vi "SwerveReverseFeedback.vi"(9 "Invert Feedback Sensor":bool, 11 "Swerve Drive Param":T1(ring)) -> ()   [LabVIEW 2016]
uses:
  Robot Global Data.vi
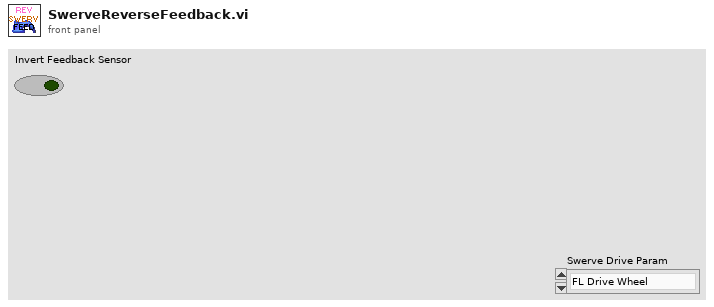
[diagram p1: front panel]
types:
  T1 = enum16{"FL Drive Wheel", "FR Drive Wheel", "RL Drive Wheel", "RR Drive Wheel", "FL Steer Wheel", "FR Steer Wheel", "RL Steer Wheel", "RR Steer Wheel"}
  T2 = typedef "WPI_DriverStationRobotMode2.ctl" = enum16{"Autonomous Disabled", "Autonomous Enabled", "Teleop Disabled", "Teleop Enabled", "Disconnected", "Finish", "Test Disabled", "Test Enabled", "Emergency Stopped"}
  T3 = typedef "WPI_CANTalonSRX_APIFeedbackSelect.ctl" = enum16{"Digital Quadrature Encoder", "Analog Potentiometer", "Analog Encoder", "Count on Quad-A (Rising-Edge)", "Count on Quad-A (Falling-Edge)", "CTR Magnetic Enc (Absolute)", "CTR Magnetic Enc (Relative)", "Pulse Width"}
  T4 = typedef "WPI_MotorControlDeviceRef.ctl" = cluster{"DeviceStatus":errorcluster, "Type":T5, "PWM":cluster{"PWM Channel":T6, "DeadBand":T7}, "CAN":cluster{"Device Number":u8, "SetOutput VI Ref":variant, "GetOutput VI Ref":variant, "Enable VI Ref":variant, "Disable VI Ref":variant, "Data":variant}, "Invert":bool}
  T5 = typedef "WPI_MotorControlType.ctl" = enum16{"PWM", "CAN"}
  T6 = typedef "FPGA_DIOPWMChannel.ctl" = enum8{"PWM 0", "PWM 1", "PWM 2", "PWM 3", "PWM 4", "PWM 5", "PWM 6", "PWM 7", "PWM 8", "PWM 9", "PWM MXP 0", "PWM MXP 1", "PWM MXP 2", "PWM MXP 3", "PWM MXP 4", "PWM MXP 5", "PWM MXP 6", "PWM MXP 7", "PWM MXP 8", "PWM MXP 9", "Invalid"}
  T7 = typedef "WPI_PWMDeadband.ctl" = cluster{"Name":string, "maxPositivePwm":i32, "minPositivePwm":i32, "centerPwm":i32, "maxNegativePwm":i32, "minNegativePwm":i32, "angularRange":u16}
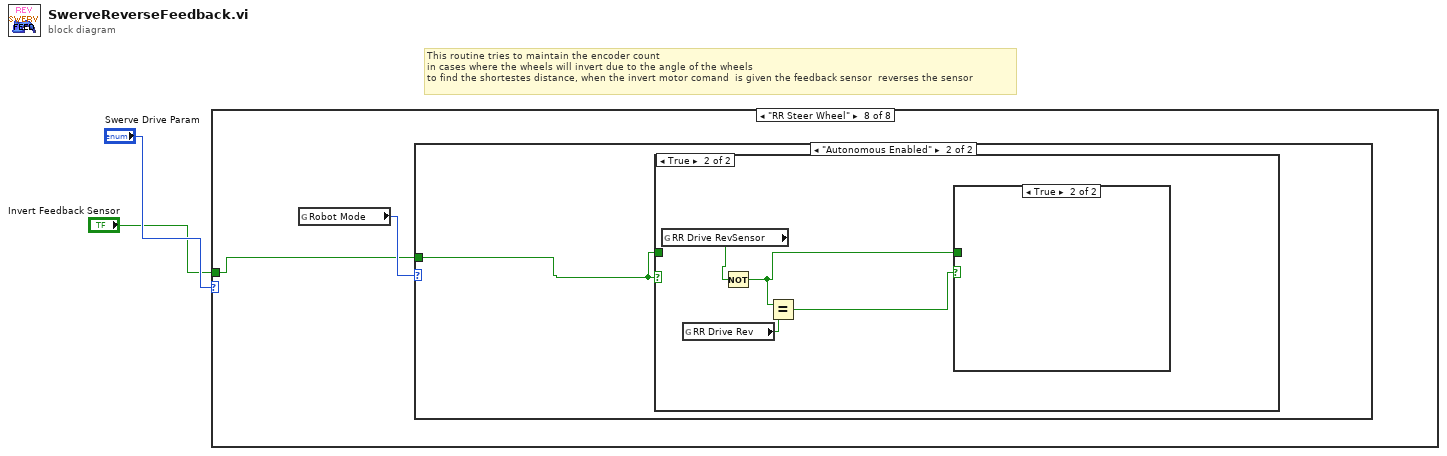
[diagram p0: block diagram]
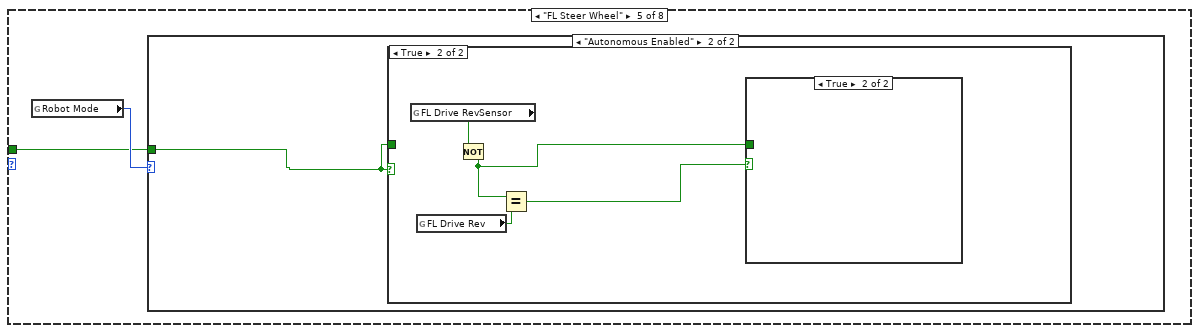
[diagram p6: hidden frame]
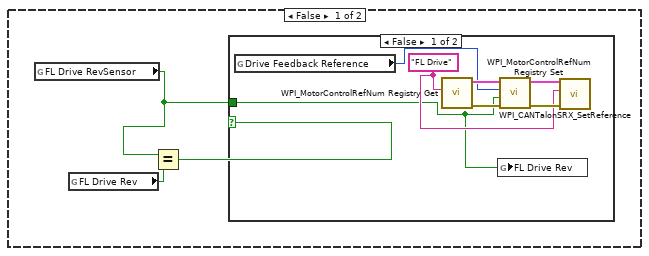
[diagram p8: hidden frame]
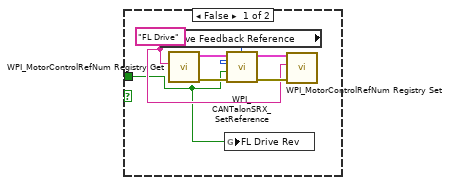
[diagram p10: hidden frame]
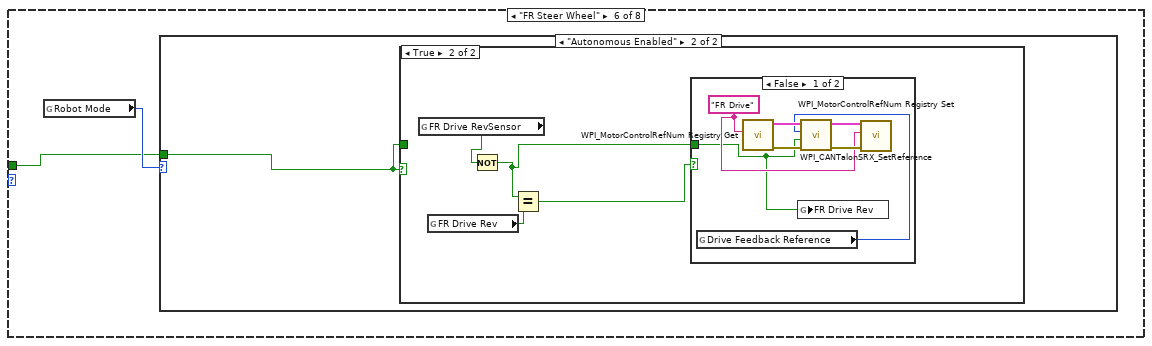
[diagram p11: hidden frame]
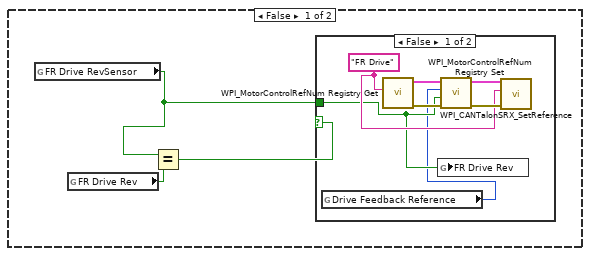
[diagram p13: hidden frame]
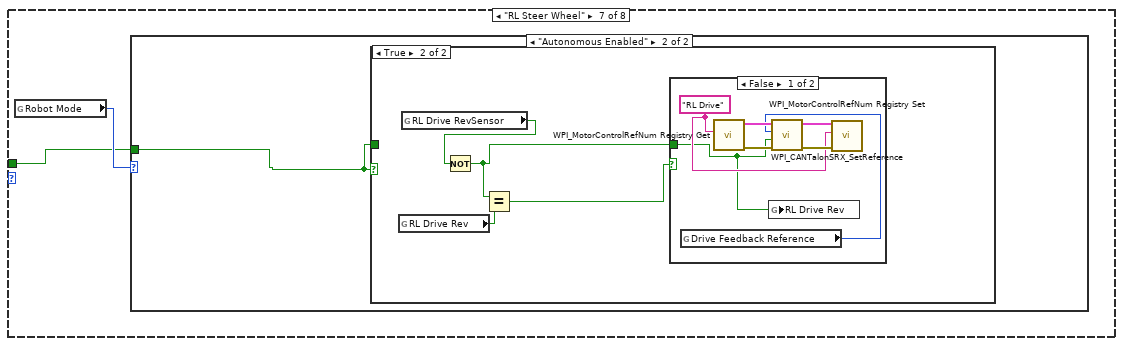
[diagram p16: hidden frame]
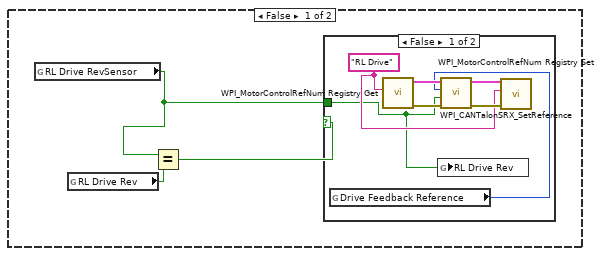
[diagram p18: hidden frame]
diagram:
  # "This routine tries to maintain the encoder count \nin cases where the wheels will invert due to the angle of the wheels \nto find the shortestes distance, when the invert motor comand  is given the feedback sensor  reverses the sensor"
  n1 = case shown="\"RR Steer Wheel\"" "Swerve Drive Param" {
    tunnel: "Invert Feedback Sensor" -> [_ _ _ _ w3 w27 w51 w75]
    frame "FL Drive Wheel", Default {
    }
    frame "FR Drive Wheel" {
    }
    frame "RL Drive Wheel" {
    }
    frame "RR Drive Wheel" {
    }
    frame "FL Steer Wheel" {
      n2 = global read "Robot Global Data.vi" "Robot Mode"() -> (w4:T2)
      n3 = case shown="\"Autonomous Enabled\"" w4 {
        tunnel: w3 -> [_ w5]
        frame "Autonomous Disabled", Default {
        }
        frame "Autonomous Enabled" {
          n4 = case shown="True" w5 {
            tunnel: w5 -> [_ _]
            frame False {
              n5 = global read "Robot Global Data.vi" "FL Drive RevSensor"() -> (w6:bool)
              n6 = global read "Robot Global Data.vi" "FL Drive Rev"() -> (w8:bool)
              n7 = Equal?(x=w6, y=w8) -> (x = y?=w7:bool)
              n8 = case shown="False" w7 {
                tunnel: w6 -> [w10 _]
                frame False {
                  w11 = "FL Drive" ("refnum name")
                  n9 = global read "Robot Global Data.vi" "Drive Feedback Reference"() -> (w9:T3)
                  n10 = call <vilib>:"WPI_MotorControlRefNum Registry Get.vi"("refnum name"=w11) -> ("error out"=w15:errorcluster, "MotorControlDevRef"=w14:T4)  [unwired: 9 in]
                  n11 = global write "Robot Global Data.vi" "FL Drive Rev"(w10) -> ()
                  n12 = call <vilib>:"WPI_CANTalonSRX_SetReference.vi"("error in (no error)"=w15, "Reverse Feedback Sensor"=w10, "Feedback Reference"=w9, "CAN Talon SRX Ref"=w14) -> ("error out"=w13:errorcluster, "CAN Talon SRX Ref"=w12:T4)  [unwired: 6 in]
                  n13 = call <vilib>:"WPI_MotorControlRefNum Registry Set.vi"("error in (no error)"=w13, "refnum name"=w11, "MotorControlDevRef"=w12) -> ()  [unwired: 7 in, 2 out]
                }
                frame True {
                }
              }
            }
            frame True {
              n14 = global read "Robot Global Data.vi" "FL Drive RevSensor"() -> (w17:bool)
              n15 = global read "Robot Global Data.vi" "FL Drive Rev"() -> (w19:bool)
              n16 = Not(x=w17) -> (.not. x?=w16:bool)
              n17 = Equal?(x=w16, y=w19) -> (x = y?=w18:bool)
              n18 = case shown="True" w18 {
                tunnel: w16 -> [w21 _]
                frame False {
                  w22 = "FL Drive" ("refnum name")
                  n19 = global read "Robot Global Data.vi" "Drive Feedback Reference"() -> (w20:T3)
                  n20 = call <vilib>:"WPI_MotorControlRefNum Registry Get.vi"("refnum name"=w22) -> ("error out"=w26:errorcluster, "MotorControlDevRef"=w25:T4)  [unwired: 9 in]
                  n21 = global write "Robot Global Data.vi" "FL Drive Rev"(w21) -> ()
                  n22 = call <vilib>:"WPI_CANTalonSRX_SetReference.vi"("error in (no error)"=w26, "Reverse Feedback Sensor"=w21, "Feedback Reference"=w20, "CAN Talon SRX Ref"=w25) -> ("error out"=w24:errorcluster, "CAN Talon SRX Ref"=w23:T4)  [unwired: 6 in]
                  n23 = call <vilib>:"WPI_MotorControlRefNum Registry Set.vi"("error in (no error)"=w24, "refnum name"=w22, "MotorControlDevRef"=w23) -> ()  [unwired: 7 in, 2 out]
                }
                frame True {
                }
              }
            }
          }
        }
      }
    }
    frame "FR Steer Wheel" {
      n24 = global read "Robot Global Data.vi" "Robot Mode"() -> (w28:T2)
      n25 = case shown="\"Autonomous Enabled\"" w28 {
        tunnel: w27 -> [_ w29]
        frame "Autonomous Disabled", Default {
        }
        frame "Autonomous Enabled" {
          n26 = case shown="True" w29 {
            tunnel: w29 -> [_ _]
            frame False {
              n27 = global read "Robot Global Data.vi" "FR Drive RevSensor"() -> (w30:bool)
              n28 = global read "Robot Global Data.vi" "FR Drive Rev"() -> (w32:bool)
              n29 = Equal?(x=w30, y=w32) -> (x = y?=w31:bool)
              n30 = case shown="False" w31 {
                tunnel: w30 -> [w34 _]
                frame False {
                  w35 = "FR Drive" ("refnum name")
                  n31 = global read "Robot Global Data.vi" "Drive Feedback Reference"() -> (w33:T3)
                  n32 = call <vilib>:"WPI_MotorControlRefNum Registry Get.vi"("refnum name"=w35) -> ("error out"=w39:errorcluster, "MotorControlDevRef"=w38:T4)  [unwired: 9 in]
                  n33 = global write "Robot Global Data.vi" "FR Drive Rev"(w34) -> ()
                  n34 = call <vilib>:"WPI_CANTalonSRX_SetReference.vi"("error in (no error)"=w39, "Reverse Feedback Sensor"=w34, "Feedback Reference"=w33, "CAN Talon SRX Ref"=w38) -> ("error out"=w37:errorcluster, "CAN Talon SRX Ref"=w36:T4)  [unwired: 6 in]
                  n35 = call <vilib>:"WPI_MotorControlRefNum Registry Set.vi"("error in (no error)"=w37, "refnum name"=w35, "MotorControlDevRef"=w36) -> ()  [unwired: 7 in, 2 out]
                }
                frame True {
                }
              }
            }
            frame True {
              n36 = global read "Robot Global Data.vi" "FR Drive RevSensor"() -> (w41:bool)
              n37 = global read "Robot Global Data.vi" "FR Drive Rev"() -> (w43:bool)
              n38 = Not(x=w41) -> (.not. x?=w40:bool)
              n39 = Equal?(x=w40, y=w43) -> (x = y?=w42:bool)
              n40 = case shown="False" w42 {
                tunnel: w40 -> [w45 _]
                frame False {
                  w46 = "FR Drive" ("refnum name")
                  n41 = global read "Robot Global Data.vi" "Drive Feedback Reference"() -> (w44:T3)
                  n42 = call <vilib>:"WPI_MotorControlRefNum Registry Get.vi"("refnum name"=w46) -> ("error out"=w50:errorcluster, "MotorControlDevRef"=w49:T4)  [unwired: 9 in]
                  n43 = global write "Robot Global Data.vi" "FR Drive Rev"(w45) -> ()
                  n44 = call <vilib>:"WPI_CANTalonSRX_SetReference.vi"("error in (no error)"=w50, "Reverse Feedback Sensor"=w45, "Feedback Reference"=w44, "CAN Talon SRX Ref"=w49) -> ("error out"=w48:errorcluster, "CAN Talon SRX Ref"=w47:T4)  [unwired: 6 in]
                  n45 = call <vilib>:"WPI_MotorControlRefNum Registry Set.vi"("error in (no error)"=w48, "refnum name"=w46, "MotorControlDevRef"=w47) -> ()  [unwired: 7 in, 2 out]
                }
                frame True {
                }
              }
            }
          }
        }
      }
    }
    frame "RL Steer Wheel" {
      n46 = global read "Robot Global Data.vi" "Robot Mode"() -> (w52:T2)
      n47 = case shown="\"Autonomous Enabled\"" w52 {
        tunnel: w51 -> [_ w53]
        frame "Autonomous Disabled", Default {
        }
        frame "Autonomous Enabled" {
          n48 = case shown="True" w53 {
            tunnel: w53 -> [_ _]
            frame False {
              n49 = global read "Robot Global Data.vi" "RL Drive RevSensor"() -> (w54:bool)
              n50 = global read "Robot Global Data.vi" "RL Drive Rev"() -> (w56:bool)
              n51 = Equal?(x=w54, y=w56) -> (x = y?=w55:bool)
              n52 = case shown="False" w55 {
                tunnel: w54 -> [w58 _]
                frame False {
                  w59 = "RL Drive" ("refnum name")
                  n53 = global read "Robot Global Data.vi" "Drive Feedback Reference"() -> (w57:T3)
                  n54 = call <vilib>:"WPI_MotorControlRefNum Registry Get.vi"("refnum name"=w59) -> ("error out"=w63:errorcluster, "MotorControlDevRef"=w62:T4)  [unwired: 9 in]
                  n55 = global write "Robot Global Data.vi" "RL Drive Rev"(w58) -> ()
                  n56 = call <vilib>:"WPI_CANTalonSRX_SetReference.vi"("error in (no error)"=w63, "Reverse Feedback Sensor"=w58, "Feedback Reference"=w57, "CAN Talon SRX Ref"=w62) -> ("error out"=w61:errorcluster, "CAN Talon SRX Ref"=w60:T4)  [unwired: 6 in]
                  n57 = call <vilib>:"WPI_MotorControlRefNum Registry Set.vi"("error in (no error)"=w61, "refnum name"=w59, "MotorControlDevRef"=w60) -> ()  [unwired: 7 in, 2 out]
                }
                frame True {
                }
              }
            }
            frame True {
              n58 = global read "Robot Global Data.vi" "RL Drive Rev"() -> (w67:bool)
              n59 = global read "Robot Global Data.vi" "RL Drive RevSensor"() -> (w65:bool)
              n60 = Not(x=w65) -> (.not. x?=w64:bool)
              n61 = Equal?(x=w64, y=w67) -> (x = y?=w66:bool)
              n62 = case shown="False" w66 {
                tunnel: w64 -> [w70 _]
                frame False {
                  w71 = "RL Drive" ("refnum name")
                  n63 = global read "Robot Global Data.vi" "Drive Feedback Reference"() -> (w68:T3)
                  n64 = call <vilib>:"WPI_MotorControlRefNum Registry Get.vi"("refnum name"=w71) -> ("error out"=w74:errorcluster, "MotorControlDevRef"=w69:T4)  [unwired: 9 in]
                  n65 = global write "Robot Global Data.vi" "RL Drive Rev"(w70) -> ()
                  n66 = call <vilib>:"WPI_CANTalonSRX_SetReference.vi"("error in (no error)"=w74, "Reverse Feedback Sensor"=w70, "Feedback Reference"=w68, "CAN Talon SRX Ref"=w69) -> ("error out"=w73:errorcluster, "CAN Talon SRX Ref"=w72:T4)  [unwired: 6 in]
                  n67 = call <vilib>:"WPI_MotorControlRefNum Registry Set.vi"("error in (no error)"=w73, "refnum name"=w71, "MotorControlDevRef"=w72) -> ()  [unwired: 7 in, 2 out]
                }
                frame True {
                }
              }
            }
          }
        }
      }
    }
    frame "RR Steer Wheel" {
      n68 = global read "Robot Global Data.vi" "Robot Mode"() -> (w76:T2)
      n69 = case shown="\"Autonomous Enabled\"" w76 {
        tunnel: w75 -> [_ w77]
        frame "Autonomous Disabled", Default {
        }
        frame "Autonomous Enabled" {
          n70 = case shown="True" w77 {
            tunnel: w77 -> [_ _]
            frame False {
              n71 = global read "Robot Global Data.vi" "RR Drive RevSensor"() -> (w78:bool)
              n72 = global read "Robot Global Data.vi" "RR Drive Rev"() -> (w80:bool)
              n73 = Equal?(x=w78, y=w80) -> (x = y?=w79:bool)
              n74 = case shown="False" w79 {
                tunnel: w78 -> [w82 _]
                frame False {
                  w83 = "RR Drive" ("refnum name")
                  n75 = global read "Robot Global Data.vi" "Drive Feedback Reference"() -> (w81:T3)
                  n76 = call <vilib>:"WPI_MotorControlRefNum Registry Get.vi"("refnum name"=w83) -> ("error out"=w87:errorcluster, "MotorControlDevRef"=w86:T4)  [unwired: 9 in]
                  n77 = global write "Robot Global Data.vi" "RR Drive Rev"(w82) -> ()
                  n78 = call <vilib>:"WPI_CANTalonSRX_SetReference.vi"("error in (no error)"=w87, "Reverse Feedback Sensor"=w82, "Feedback Reference"=w81, "CAN Talon SRX Ref"=w86) -> ("error out"=w85:errorcluster, "CAN Talon SRX Ref"=w84:T4)  [unwired: 6 in]
                  n79 = call <vilib>:"WPI_MotorControlRefNum Registry Set.vi"("error in (no error)"=w85, "refnum name"=w83, "MotorControlDevRef"=w84) -> ()  [unwired: 7 in, 2 out]
                }
                frame True {
                }
              }
            }
            frame True {
              n80 = global read "Robot Global Data.vi" "RR Drive RevSensor"() -> (w89:bool)
              n81 = global read "Robot Global Data.vi" "RR Drive Rev"() -> (w91:bool)
              n82 = Not(x=w89) -> (.not. x?=w88:bool)
              n83 = Equal?(x=w88, y=w91) -> (x = y?=w90:bool)
              n84 = case shown="True" w90 {
                tunnel: w88 -> [w93 _]
                frame False {
                  w94 = "RR Drive" ("refnum name")
                  n85 = global read "Robot Global Data.vi" "Drive Feedback Reference"() -> (w92:T3)
                  n86 = call <vilib>:"WPI_MotorControlRefNum Registry Get.vi"("refnum name"=w94) -> ("error out"=w98:errorcluster, "MotorControlDevRef"=w97:T4)  [unwired: 9 in]
                  n87 = global write "Robot Global Data.vi" "RR Drive Rev"(w93) -> ()
                  n88 = call <vilib>:"WPI_CANTalonSRX_SetReference.vi"("error in (no error)"=w98, "Reverse Feedback Sensor"=w93, "Feedback Reference"=w92, "CAN Talon SRX Ref"=w97) -> ("error out"=w96:errorcluster, "CAN Talon SRX Ref"=w95:T4)  [unwired: 6 in]
                  n89 = call <vilib>:"WPI_MotorControlRefNum Registry Set.vi"("error in (no error)"=w96, "refnum name"=w94, "MotorControlDevRef"=w95) -> ()  [unwired: 7 in, 2 out]
                }
                frame True {
                }
              }
            }
          }
        }
      }
    }
  }
